vi "GetUser.vi"(8 "error in":errorcluster, 11 "UserComment in":refnum<class "UserComment.lvclass">) -> (0 "error out":errorcluster, 2 "User":string, 3 "UserComment out":refnum<class "UserComment.lvclass">)   [LabVIEW 2021, in "ProligentXMLGenerator.lvlib" / "UserComment.lvclass"]
uses:
  UserComment.lvclass
  UserComment.lvclass/UserComment.ctl
  Base/NonEmptyString_255/NonEmptyString_255.lvclass
  Base/Attribute/Attribute.lvclass
  C:/Projects/proligent-xml-generator-labview/src/ProligentXMLGenerator/Base/NonEmptyString/NonEmptyString.lvclass
  C:/Projects/proligent-xml-generator-labview/src/ProligentXMLGenerator/Base/String/String.lvclass
  C:/Projects/proligent-xml-generator-labview/src/ProligentXMLGenerator/Base/Attribute/Attribute.lvclass
  C:/Projects/proligent-xml-generator-labview/src/ProligentXMLGenerator/Base/NonEmptyString_255/NonEmptyString_255.lvclass
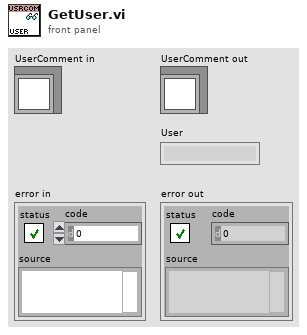
[diagram p1: front panel]
types:
  T1 = typedef "ProligentXMLGenerator.lvlib/UserComment.lvclass/Data.ctl" = cluster{"Name":string, "Comment":refnum<class "NonNullableString_TruncateAt_255.lvclass">, "User":refnum<class "NonEmptyString_255.lvclass">, "Time":refnum<class "DateTime.lvclass">}
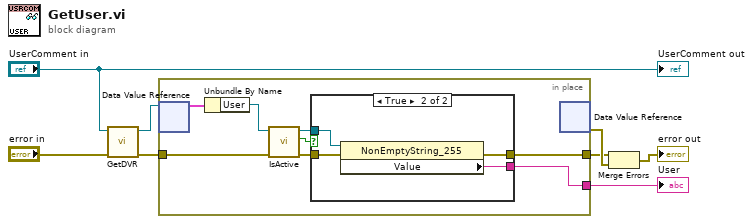
[diagram p0: block diagram]
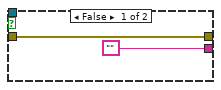
[diagram p2: hidden frame]
diagram:
  n1 = call "GetDVR.vi"("error in"="error in", "UserComment"="UserComment in") -> ("error out"=w4:errorcluster, "DVRReference"=w7:refnum<data-value>)  [unwired: 8 in]
  n2 = in-place "In Place Element Structure" {
    in-place-border: w4 -> [w12]
    in-place-border: [w15] -> w3
    in-place-border: [w14] -> w1
    n3 = in-place-dvr #1(w7) -> (w16:T1)  [unwired: 1 out]
    n4 = Unbundle By Name(w16) -> ("User"=w13:refnum<class "NonEmptyString_255.lvclass">)
    n5 = call "IsActive.vi"("error in"=w12, "Attribute in"=w13) -> ("error out"=w10:errorcluster, "IsActive"=w9:bool, "Attribute in"=w11:refnum<class "NonEmptyString_255.lvclass">)  [unwired: 7 in]
    n6 = case shown="True" w9 {
      tunnel: [w18 w22] -> w15
      tunnel: ["" ("Empty String Constant") w21] -> w14
      tunnel: w11 -> [_ w20]
      tunnel: w10 -> [w18 w19]
      frame False {
      }
      frame True {
        n7 = property on="Property Node" class="NonEmptyString_255"(reference=w20, error in=w19) -> (error out=w22:errorcluster, "Value"=w21:string)  [unwired: 1 out]
      }
    }
    n8 = in-place-dvr #1() -> (w8:errorcluster)  [unwired: 1 in, 1 out]
  }
  "User" <- w1
  n9 = Merge Errors(w3, w8) -> (→"error out":errorcluster)
  "UserComment out" <- "UserComment in"
